vi "Initialize Instrument.vi"(8 "error in (no error)":errorcluster, 10 "Reset":bool, 11 "E364x in":refnum<class "E364x.lvclass">) -> (0 "error out":errorcluster, 3 "E364x out":refnum<class "E364x.lvclass">)   [LabVIEW 2020, in "E364x.lvclass"]
uses:
  E364x.lvclass
  C:/Sandbox/Git_Sandbox/WiSpry Test Framework source code (LV20)/WiSpry Test Framework/Instruments/Instrument.lvclass
  Instrument.lvclass/Instrument.ctl
  Power Supply.lvclass
  Instrument.lvclass
  <instrlib>/Agilent E364X Series/Agilent E364X Series.lvlib
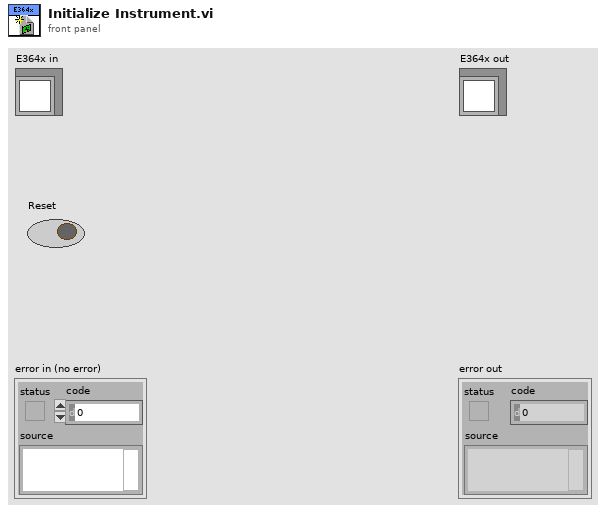
[diagram p1: front panel]
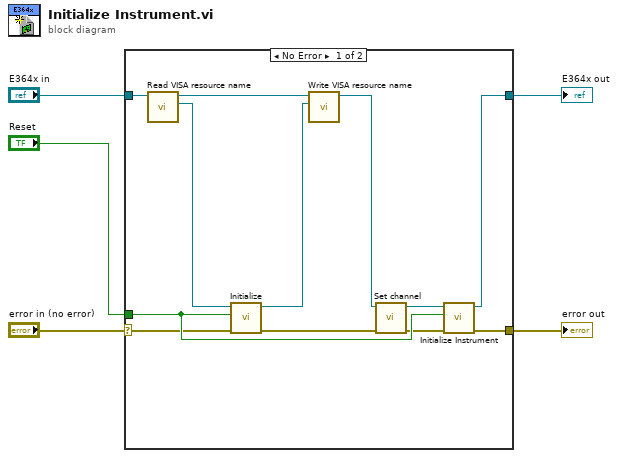
[diagram p0: block diagram]
diagram:
  n1 = case shown="No Error" "error in (no error)" {
    selector: "error in (no error)" -> [w6 w19]
    tunnel: [w8 w19] -> w5
    tunnel: [w9 w18] -> w4
    tunnel: "Reset" -> [w14 _]
    tunnel: "E364x in" -> [w13 w18]
    frame No Error {
      n2 = call "Read VISA resource name.vi"("Instrument in"=w13) -> ("VISA resource name"=w17:refnum<visa-resource-name>, "Instrument out"=w16:refnum<class "E364x.lvclass">)  [unwired: 9 in]
      n3 = call <instrlib>:"Initialize.vi"("error in (no error)"=w6, "Reset Device (T: Reset)"=w14, "VISA resource name"=w17) -> ("error out"=w7:errorcluster, "VISA resource name out"=w15:refnum<visa-resource-name>)  [unwired: 7 in]
      n4 = call "Write VISA resource name.vi"("VISA resource name"=w15, "Instrument in"=w16) -> ("Instrument out"=w10:refnum<class "E364x.lvclass">)  [unwired: 9 in]
      n5 = call "Set channel.vi"("error in (no error)"=w7, "E364x in"=w10) -> ("error out"=w12:errorcluster, "E364x out"=w11:refnum<class "E364x.lvclass">)  [unwired: 7 in, 1 out]
      n6 = call-parent "Initialize Instrument.vi"("error in (no error)"=w12, "Reset"=w14, "Power Supply in"=w11) -> ("error out"=w8:errorcluster, "Power Supply out"=w9:refnum<class "E364x.lvclass">)  [unwired: 7 in]
    }
    frame Error {
    }
  }
  "error out" <- w5
  "E364x out" <- w4
